vi "IsValidHexCode.vi"(11 "Input String":string) -> (3 "Valid?":bool)   [LabVIEW 2020]
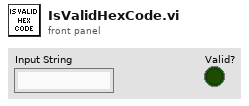
[diagram p1: front panel]
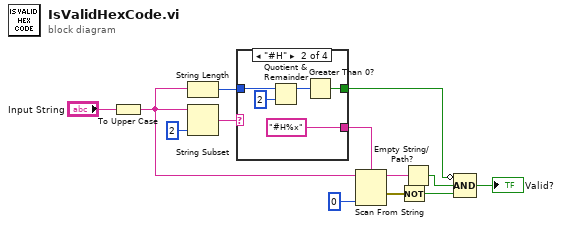
[diagram p0: block diagram]
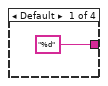
[diagram p2: hidden frame]
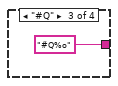
[diagram p3: hidden frame]
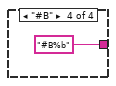
[diagram p4: hidden frame]
diagram:
  n1 = To Upper Case(1:"Input String") -> (0:w3:string)
  n2 = String Length(string=w3) -> (length=w2:i32)
  n3 = String Subset(string=w3, length (rest)=2 ("length (rest)")) -> (substring=w11:string)  [unwired: 1 in]
  n4 = case shown="\"#H\"" w11 {
    tunnel: ["%d" ("format string") "#H%x" ("format string") "#Q%o" ("format string") "#B%b" ("format string")] -> w10
    tunnel: w2 -> [_ w18 _ _]
    tunnel: [_ w15 _ _] -> w1
    frame Default {
    }
    frame "#H" {
      n5 = Quotient & Remainder(x=w18, y=2) -> (x-y*floor(x/y)=w16:i32)  [unwired: 1 out]
      n6 = Greater Than 0?(x=w16) -> (x > 0?=w15:bool)
    }
    frame "#Q" {
    }
    frame "#B" {
    }
  }
  n7 = Scan From String(format string=w10, input string=w3, default 1=0) -> (remaining string=w7:string, error out=w9:errorcluster)  [unwired: 3 in, 1 out]
  n8 = Not(x=w9) -> (.not. x?=w6:bool)
  n9 = Empty String/Path?(string/path=w7) -> (empty?=w5:bool)
  n10 = Compound Arithmetic op=AND(invert w1, w5, w6) -> (→"Valid?":bool)
